vi "ReadMessageCluster.vi"(6 "timeout in ms (-1)":i32=-1, 8 "error in":errorcluster, 11 "message ref in":refnum<class "CLM_PriorityLocalMessage.lvclass">) -> (0 "error out":errorcluster, 2 "message":T1, 3 "message ref out":refnum<class "CLM_PriorityLocalMessage.lvclass">, 4 "timed out?":bool, 5 "priority":i32)   [LabVIEW 2013, in "CLM_PriorityLocalMessage.lvclass"]
uses:
  CLM_PriorityLocalMessage.lvclass
  LocalMessage/Message.ctl
  CLM_PriorityLocalMessage.lvclass/CLM_PriorityLocalMessage.ctl
  LocalMessage_Queue/CLM_LocalMessage_Queue.lvclass/CLM_LocalMessage_Queue.ctl
  LocalMessage_Queue/CLM_LocalMessage_Queue.lvclass
  LocalMessage/CLM_LocalMessage.lvclass
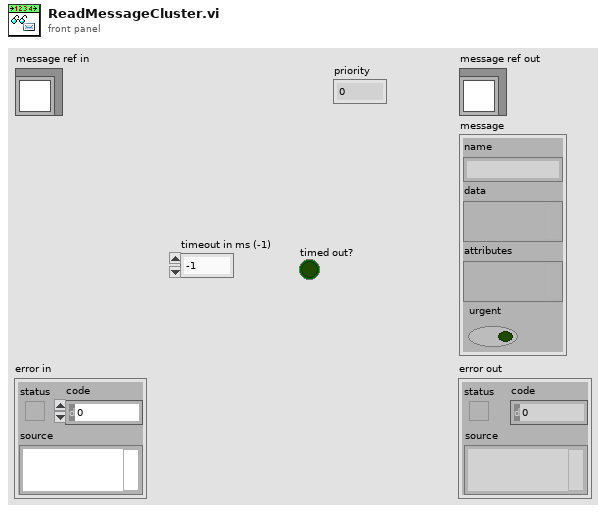
[diagram p1: front panel]
types:
  T1 = typedef "CLM_LocalMessage.lvclass/Message.ctl" = cluster{"name":string, "data":variant, "attributes":variant, "urgent":bool}
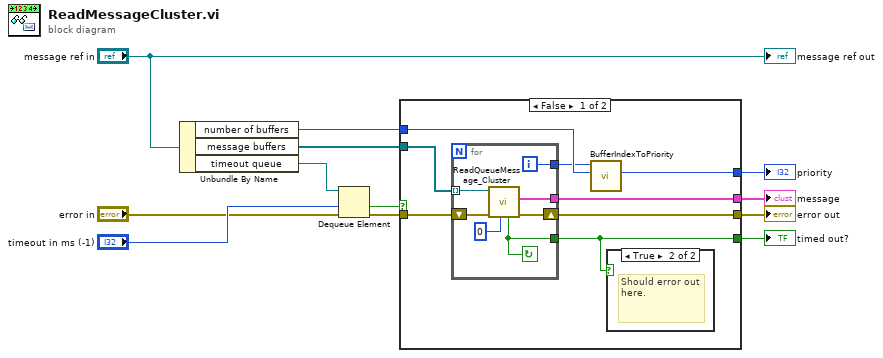
[diagram p0: block diagram]
diagram:
  n1 = Unbundle By Name("message ref in") -> ("number of buffers"=w1:i32, "message buffers"=w8:refnum<class "CLM_LocalMessage_Queue.lvclass">[], "timeout queue"=w7:refnum<queue>)
  n2 = Dequeue Element(queue=w7, timeout in ms (-1)="timeout in ms (-1)", error in (no error)="error in") -> (timed out?=w10:bool, error out=w9:errorcluster)  [unwired: 2 out]
  n3 = case shown="False" w10 {
    selector: w10 -> [_ w29]
    tunnel: w9 -> [w20 w28]
    tunnel: w8 -> [w19 _]
    tunnel: [w16 w29] -> w6
    tunnel: [w18 w28] -> w5
    tunnel: [w17 _] -> w4
    tunnel: [w13 _] -> w2
    tunnel: w1 -> [w15 _]
    frame False {
      n4 = for {
        tunnel: w19 -> [w27] mode=indexing
        shift-right: [w26] -> w18
        shift-left: w20 -> [w25]
        tunnel: [w23] -> w17
        tunnel: [w22] -> w16
        tunnel: [w21] -> w14
        i -> [w21]
        stop <- w22 continue-if-true
        n5 = call "ReadQueueMessage_Cluster.vi"("timeout in ms (-1)"=0, "error in"=w25, "message ref in"=w27) -> ("error out"=w26:errorcluster, "message"=w23:T1, "timed out?"=w22:bool)  [unwired: 5 in, 1 out]
      }
      n6 = call "BufferIndexToPriority.vi"("number of buffers"=w15, "buffer index"=w14) -> ("priority"=w13:i32)  [unwired: 6 in, 3 out]
      n7 = case shown="True" w16 {
        frame False {
        }
        frame True {
          # "Should error out here."
        }
      }
    }
    frame True {
    }
  }
  "error out" <- w5
  "timed out?" <- w6
  "message" <- w4
  "priority" <- w2
  "message ref out" <- "message ref in"
